vi "Process.vi"(2 "reference fpga":refnum<class "niUSRP Reference FPGA v1.lvclass">) -> ()   [LabVIEW 2025, in "niUSRP Reference FPGA v1.lvclass"]
uses:
  niUSRP Reference FPGA v1.lvclass
  niUSRP Reference FPGA v1.lvclass/niUSRP Reference FPGA v1.ctl
  <instrlib>/_niInstr/Instruction Framework/v1/FPGA/Top Level Bus/Register Configuration/Register Configuration.lvclass
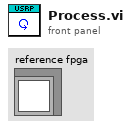
[diagram p1: front panel]
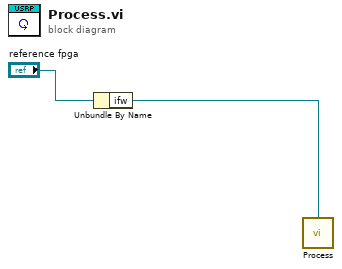
[diagram p0: block diagram]
diagram:
  n1 = Unbundle By Name("reference fpga") -> ("ifw"=w1:refnum<class "Register Configuration.lvclass">)
  n2 = call-dynamic "Process.vi"("register configuration"=w1) -> ()  [unwired: 15 in]
